vi "Create File for Conveyor and Shooter SS.vi"() -> (2 "File Reference Out":refnum<file>)   [LabVIEW 2016]
uses:
  Global Variables/Folder Names.vi
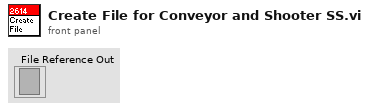
[diagram p1: front panel]
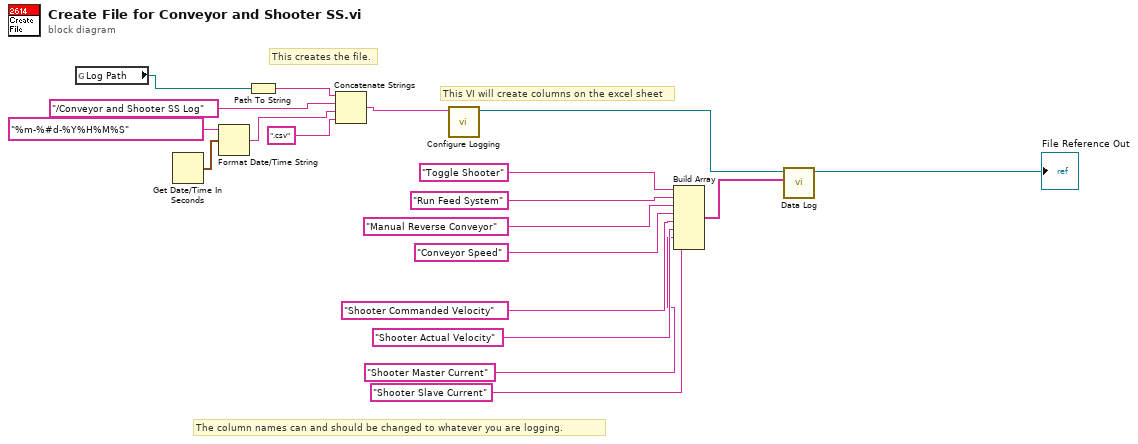
[diagram p0: block diagram]
diagram:
  # "The column names can and should be changed to whatever you are logging."
  # "This VI will create columns on the excel sheet"
  # "This creates the file."
  n1 = global read "Folder Names.vi" "Log Path"() -> (w17:path)
  n2 = Get Date/Time In Seconds() -> (seconds since 1Jan1904=w13:timestamp)
  n3 = Format Date/Time String(time format string (%c)="%m-%#d-%Y%H%M%S", seconds (now)=w13) -> (date/time string=w11:string)  [unwired: 1 in]
  n4 = Path To String(path=w17) -> (string=w16:string)
  n5 = Concatenate Strings(w16, "/Conveyor and Shooter SS Log" ("string"), w11, ".csv" ("string")) -> (w18:string)
  n6 = call "Configure Logging.vi"("File Path/File Name"=w18) -> ("refnum out"=w15:refnum<file>)  [unwired: 10 in]
  n7 = Build Array("Toggle Shooter" ("File Path/File Name"), "Run Feed System" ("element"), "Manual Reverse Conveyor" ("element"), "Conveyor Speed" ("File Path/File Name"), "Shooter Commanded Velocity" ("element"), "Shooter Actual Velocity" ("element"), "Shooter Master Current" ("element"), "Shooter Slave Current" ("element")) -> (w4:string[])
  n8 = call "Data Log.vi"("Data In"=w4, "File Reference In"=w15) -> ("File Reference Out"=→"File Reference Out":refnum<file>)  [unwired: 9 in]
